vi "RateLimiter.vi"(10 "Rate":dbl, 11 "Input":dbl(slide) scale=-1.0..1.0) -> (3 "Output":dbl(slide) scale=-1.0..1.0)   [LabVIEW 2016]
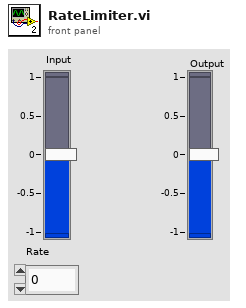
[diagram p1: front panel]
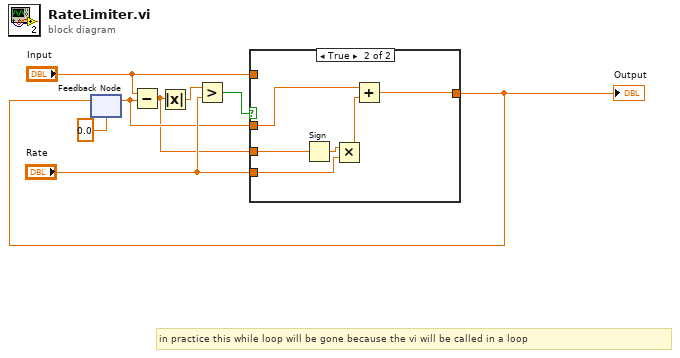
[diagram p0: block diagram]
diagram:
  # "in practice this while loop will be gone because the vi will be called in a loop"
  n1 = feedback #1(0.0) -> (w4:dbl)
  n2 = Subtract(x="Input", y=w4) -> (x-y=w1:dbl)
  n3 = Absolute Value(x=w1) -> (abs(x)=w6:dbl)
  n4 = Greater?(x=w6, y="Rate") -> (0:w7:bool)
  n5 = case shown="True" w7 {
    tunnel: "Rate" -> [_ w13]
    tunnel: "Input" -> [w9 _]
    tunnel: [w9 w15] -> w3
    tunnel: w4 -> [_ w11]
    tunnel: w1 -> [_ w10]
    frame False {
    }
    frame True {
      n6 = Sign(1:w10) -> (0:w14:dbl)
      n7 = Multiply(x=w14, y=w13) -> (x*y=w12:dbl)
      n8 = Add(x=w11, y=w12) -> (x+y=w15:dbl)
    }
  }
  "Output" <- w3
  n9 = feedback-in #1(w3) -> ()
